vi "Calculate Frequency (Normal Mode).vi"(9 "Clock Divisor":u32, 10 "TOP":dbl, 11 "Base Clock Frequency (Hz)":dbl) -> (3 "Frequency (Hz)":dbl format="%#.2f")   [LabVIEW 2021]
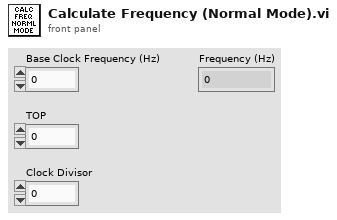
[diagram p1: front panel]
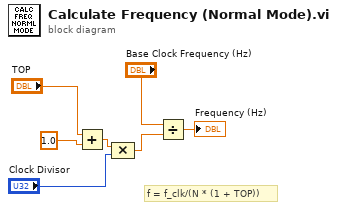
[diagram p0: block diagram]
diagram:
  # "f = f_clk/(N * (1 + TOP))"
  n1 = Add(x="TOP", y=1.0 ("value")) -> (x+y=w5:dbl)
  n2 = Compound Arithmetic op=MULTIPLY(w5, "Clock Divisor") -> (w2:dbl)
  n3 = Divide(x="Base Clock Frequency (Hz)", y=w2) -> (x/y=→"Frequency (Hz)":dbl)
